vi "sendTCPString.vi"(9 "imput string":string, 11 "connection ID":refnum<k5>) -> ()   [LabVIEW 2011]
panel:
  in  "1st Error to Convert":i32(ring) items=["No Error", "Argument Error", "Memory Full", "Out of Zone", "End of File", "File Already Open", "Generic File IO Error", "File Not Found", "File Permission Error", "Disk Full", "Duplicate Path", "Too Many Files Open", "Not Enabled", "Resource File Not Found", "Cannot Add Resource", "Resource Not Found", "Image Not Found", "Image Memory Error", "Pen Does Not Exist", "Config Bad Type", "Config Token Not Found", "Config Parse Error", "Config Memory Error", "Bad External Code Format", "Bad External Code Offset", "External Code Not Present", "Null Window", "Destroy Window Mixup", "Null Menu", "Print Aborted", "Bad Print Record", "Print Driver Error", "Windows Error During Print", "Memory Error During Print", "Print Dialog Error", "Generic Print Error", "Invalid Device Refnum", "Device Not Found", "Device Parameter Error", "Device Unit Error", "Can't Open Device", "Device Call Aborted", "Generic Error", "Cancelled By User", "Object ID Too Low", "Object ID Too High", "Object Not In Heap", "Unknown Heap", "Bad DefProc ID", "DefProc Not In Table", "Message Out Of Range", "Null Method", "Unknown Message", "Manager Call Not Supported", "Bad address", "Connection In progress", "Connection timed out", "Connection is already in progress", "Network attribute not supported", "Network error", "Address in use", "System out of memory", "Connection aborted", "Connection refused", "Connection is not connected", "Connection is already connected", "Connection closed", "Initialize error (interapplication manager)", "Bad occurrence", "Wait on unbound occurrence handler", "Occurrence queue overflow", "Bad path", "Semaphore not signaled", "Unrecognized type (interapplication manager)"]
  in  "error in":errorcluster
  out "error out 2":errorcluster
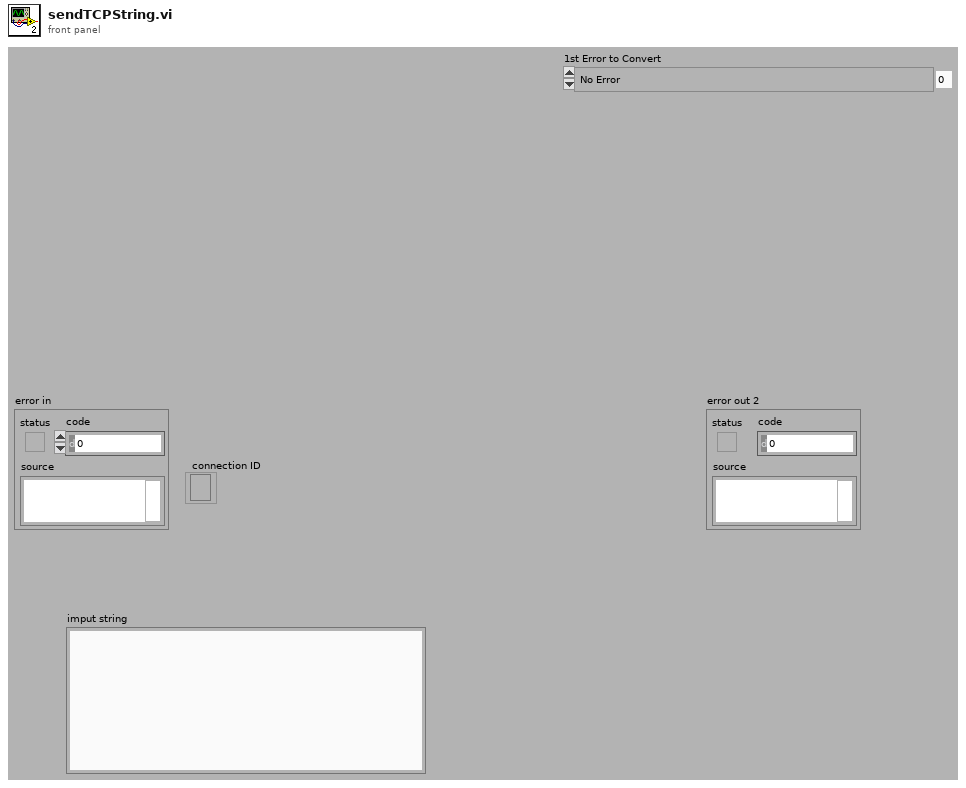
[diagram p1: front panel]
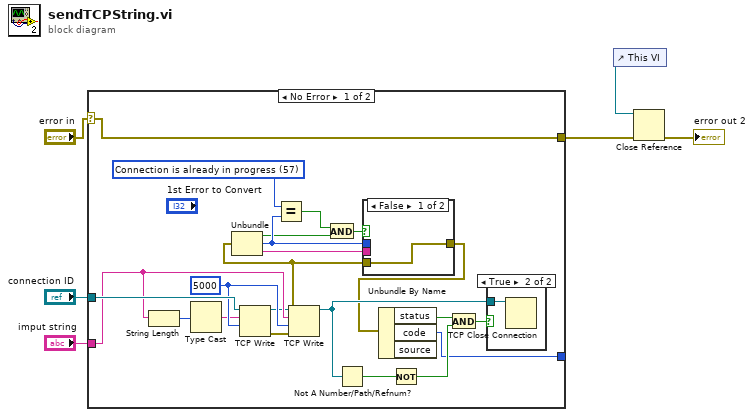
[diagram p0: block diagram]
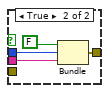
[diagram p2: hidden frame]
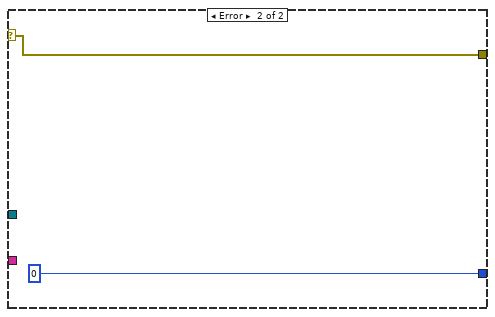
[diagram p4: hidden frame]
diagram:
  n1 = case shown="No Error" "error in" {
    selector: "error in" -> [w7 w35]
    tunnel: "connection ID" -> [w28 _]
    tunnel: "imput string" -> [w22 _]
    tunnel: [w7 w35] -> w4
    tunnel: [w16 0 ("code")] -> _
    frame No Error {
      w10 = 57 items=["No Error", "Argument Error", "Memory Full", "Out of Zone", "End of File", "File Already Open", "Generic File IO Error", "File Not Found", "File Permission Error", "Disk Full", "Duplicate Path", "Too Many Files Open", "Not Enabled", "Resource File Not Found", "Cannot Add Resource", "Resource Not Found", "Image Not Found", "Image Memory Error", "Pen Does Not Exist", "Config Bad Type", "Config Token Not Found", "Config Parse Error", "Config Memory Error", "Bad External Code Format", "Bad External Code Offset", "External Code Not Present", "Null Window", "Destroy Window Mixup", "Null Menu", "Print Aborted", "Bad Print Record", "Print Driver Error", "Windows Error During Print", "Memory Error During Print", "Print Dialog Error", "Generic Print Error", "Invalid Device Refnum", "Device Not Found", "Device Parameter Error", "Device Unit Error", "Can't Open Device", "Device Call Aborted", "Generic Error", "Cancelled By User", "Object ID Too Low", "Object ID Too High", "Object Not In Heap", "Unknown Heap", "Bad DefProc ID", "DefProc Not In Table", "Message Out Of Range", "Null Method", "Unknown Message", "Manager Call Not Supported", "Bad address", "Connection In progress", "Connection timed out", "Connection is already in progress", "Network attribute not supported", "Network error", "Address in use", "System out of memory", "Connection aborted", "Connection refused", "Connection is not connected", "Connection is already connected", "Connection closed", "Initialize error (interapplication manager)", "Bad occurrence", "Wait on unbound occurrence handler", "Occurrence queue overflow", "Bad path", "Semaphore not signaled", "Unrecognized type (interapplication manager)"] ("1st Error to Convert")
      w21 = 5000 ("timeout ms (25000)")
      n2 = String Length(string=w22) -> (length=w18:i32)
      n3 = Type Cast(x=w18) -> (*(type *) &x=w17:string)  [unwired: 1 in]
      n4 = TCP Write(connection ID=w28, data in=w17, 9:w21) -> (connection ID out=w20:refnum<k5>, error out=w19:errorcluster)  [unwired: 1 in, 1 out]
      n5 = TCP Write(connection ID=w20, data in=w22, error in (no error)=w19, 9:w21) -> (connection ID out=w27:refnum<k5>, error out=w9:errorcluster)  [unwired: 1 out]
      n6 = Unbundle(w9) -> ("status"=w11:bool, "code"=w14:i32, "source"=w13:string)
      n7 = Equal?(x=w10, y=w14) -> (x = y?=w15:bool)
      n8 = And(x=w15, y=w11) -> (x .and. y?=w12:bool)
      n9 = Not A Number/Path/Refnum?(number/path/refnum=w27) -> (NaN/Path/Refnum?=w26:bool)
      n10 = case shown="False" w12 {
        tunnel: w9 -> [w29 _]
        tunnel: [w29 w33] -> w8
        tunnel: w13 -> [_ w32]
        tunnel: w14 -> [_ w31]
        frame False {
        }
        frame True {
          n11 = Bundle(FALSE, "code"=w31, "source"=w32) -> (w33:cluster{bool, "code":i32, "source":string})  [unwired: 1 in]
        }
      }
      n12 = Unbundle By Name(w8) -> ("status"=w25:bool, "code"=w16:i32)  [unwired: 1 out]
      n13 = Not(x=w26) -> (.not. x?=w24:bool)
      n14 = And(x=w25, y=w24) -> (x .and. y?=w23:bool)
      n15 = case shown="True" w23 {
        tunnel: w27 -> [_ w34]
        frame False {
        }
        frame True {
          n16 = TCP Close Connection(connection ID=w34) -> ()  [unwired: 2 in, 2 out]
        }
      }
    }
    frame Error {
    }
  }
  n17 = control-ref of="This VI"() -> (w2:refnum<vi>)
  n18 = Close Reference(reference=w2, error in (no error)=w4) -> (error out=→"error out 2":errorcluster)
